vi "FGV Post Processing.vi"(4 "reprocessing index for filname":i32, 5 "LIN/EPA Refs Array":refnum<vi>[](array[refnum]), 6 "Aktion":T7, 7 "Refs Cluster":T3, 8 "error in (no error)":errorcluster caption="Fehler (Eingang, kein Fehler)", 9 "active Index Cluster in":T1, 10 "filenemas Cluster":T6, 11 "SpanInletClusterArray in":T8[](array[typedef]) {"zusätzliche Zeitdauer Erster Punkt" min=30 step=1 format="%#_5g"; "Zeitdauer Stufen" format="%#_5g"; "Max Fehler" format="%#_5g"; "Anzahl Stufen" format="%#_5g"; "Komponenten"."Komponente 5"."Komponente:" items=["NO (350,3000) LP 191C", "NO2 (150) LP 191C (1of2)", "NO2 (2000) LP 191C (2of2)", "N2O (300) LP 191C (1of2)", "NH3 (300) LP 191C (1of2)", "NH3 (900,3000) LP 191C (2of2)", "HNCO (400) 191C", "H2O% (30) LP 191C", "Formaldehyde (70,500) LP 191C", "CO2 low% (4) LP 191C (2of2)", "CO2% (20) LP 191C (1of2)", "CO (700) LP 191C (1of3)", "CO% (1) LP 191C (2of3)", "Propylene (1000) LP 191C", "Aromatic HC C7 (500) LP 191C", "Ethylene (1000) LP 191C", "CH4 (250) LP 191C (1of2)", "CH4 (5000) LP 191C (2of2)", "Ethane (1000) LP 191C", "Acetylene (1000) LP 191C", "HNO2 (20) 191C", "MeOH (1000) 191C", "CO% (10) LP 191C (3of3)", "Formic Acid (100) 191C", "SO2 (500) LP 191C", "Acetaldehyde (1000) LP 191C", "COS (100) LP 191C", "1,3 butadiene (100) LP 191C", "Oil as Octane (200) LP 191C", "N2O (1000) LP 191C (2of2)", "Propane (200) LP 191C", "NO2 autorange (2000)", "CO autorange (100000)", "CH4 autorange (5000)", "NH3 autorange (3000)", "Temp. Gascell", "Pressure Gascell", "sBeam@2500"]; "Komponenten"."Komponente 5"."Konzentration IST" format="%#.4f"; "Komponenten"."Komponente 5"."Genauigkeit" format="%#.1f"; "Komponenten"."Komponente 4"."Komponente:" items=["NO (350,3000) LP 191C", "NO2 (150) LP 191C (1of2)", "NO2 (2000) LP 191C (2of2)", "N2O (300) LP 191C (1of2)", "NH3 (300) LP 191C (1of2)", "NH3 (900,3000) LP 191C (2of2)", "HNCO (400) 191C", "H2O% (30) LP 191C", "Formaldehyde (70,500) LP 191C", "CO2 low% (4) LP 191C (2of2)", "CO2% (20) LP 191C (1of2)", "CO (700) LP 191C (1of3)", "CO% (1) LP 191C (2of3)", "Propylene (1000) LP 191C", "Aromatic HC C7 (500) LP 191C", "Ethylene (1000) LP 191C", "CH4 (250) LP 191C (1of2)", "CH4 (5000) LP 191C (2of2)", "Ethane (1000) LP 191C", "Acetylene (1000) LP 191C", "HNO2 (20) 191C", "MeOH (1000) 191C", "CO% (10) LP 191C (3of3)", "Formic Acid (100) 191C", "SO2 (500) LP 191C", "Acetaldehyde (1000) LP 191C", "COS (100) LP 191C", "1,3 butadiene (100) LP 191C", "Oil as Octane (200) LP 191C", "N2O (1000) LP 191C (2of2)", "Propane (200) LP 191C", "NO2 autorange (2000)", "CO autorange (100000)", "CH4 autorange (5000)", "NH3 autorange (3000)", "Temp. Gascell", "Pressure Gascell", "sBeam@2500"]; "Komponenten"."Komponente 4"."Konzentration IST" format="%#.4f"; "Komponenten"."Komponente 4"."Genauigkeit" format="%#.1f"; "Komponenten"."Komponente 3"."Komponente:" items=["NO (350,3000) LP 191C", "NO2 (150) LP 191C (1of2)", "NO2 (2000) LP 191C (2of2)", "N2O (300) LP 191C (1of2)", "NH3 (300) LP 191C (1of2)", "NH3 (900,3000) LP 191C (2of2)", "HNCO (400) 191C", "H2O% (30) LP 191C", "Formaldehyde (70,500) LP 191C", "CO2 low% (4) LP 191C (2of2)", "CO2% (20) LP 191C (1of2)", "CO (700) LP 191C (1of3)", "CO% (1) LP 191C (2of3)", "Propylene (1000) LP 191C", "Aromatic HC C7 (500) LP 191C", "Ethylene (1000) LP 191C", "CH4 (250) LP 191C (1of2)", "CH4 (5000) LP 191C (2of2)", "Ethane (1000) LP 191C", "Acetylene (1000) LP 191C", "HNO2 (20) 191C", "MeOH (1000) 191C", "CO% (10) LP 191C (3of3)", "Formic Acid (100) 191C", "SO2 (500) LP 191C", "Acetaldehyde (1000) LP 191C", "COS (100) LP 191C", "1,3 butadiene (100) LP 191C", "Oil as Octane (200) LP 191C", "N2O (1000) LP 191C (2of2)", "Propane (200) LP 191C", "NO2 autorange (2000)", "CO autorange (100000)", "CH4 autorange (5000)", "NH3 autorange (3000)", "Temp. Gascell", "Pressure Gascell", "sBeam@2500"]; "Komponenten"."Komponente 3"."Konzentration IST" format="%#.4f"; "Komponenten"."Komponente 3"."Genauigkeit" format="%#.1f"; "Komponenten"."Komponente 2"."Komponente:" items=["NO (350,3000) LP 191C", "NO2 (150) LP 191C (1of2)", "NO2 (2000) LP 191C (2of2)", "N2O (300) LP 191C (1of2)", "NH3 (300) LP 191C (1of2)", "NH3 (900,3000) LP 191C (2of2)", "HNCO (400) 191C", "H2O% (30) LP 191C", "Formaldehyde (70,500) LP 191C", "CO2 low% (4) LP 191C (2of2)", "CO2% (20) LP 191C (1of2)", "CO (700) LP 191C (1of3)", "CO% (1) LP 191C (2of3)", "Propylene (1000) LP 191C", "Aromatic HC C7 (500) LP 191C", "Ethylene (1000) LP 191C", "CH4 (250) LP 191C (1of2)", "CH4 (5000) LP 191C (2of2)", "Ethane (1000) LP 191C", "Acetylene (1000) LP 191C", "HNO2 (20) 191C", "MeOH (1000) 191C", "CO% (10) LP 191C (3of3)", "Formic Acid (100) 191C", "SO2 (500) LP 191C", "Acetaldehyde (1000) LP 191C", "COS (100) LP 191C", "1,3 butadiene (100) LP 191C", "Oil as Octane (200) LP 191C", "N2O (1000) LP 191C (2of2)", "Propane (200) LP 191C", "NO2 autorange (2000)", "CO autorange (100000)", "CH4 autorange (5000)", "NH3 autorange (3000)", "Temp. Gascell", "Pressure Gascell", "sBeam@2500"]; "Komponenten"."Komponente 2"."Konzentration IST" format="%#.4f"; "Komponenten"."Komponente 2"."Genauigkeit" format="%#.1f"; "Komponenten"."Komponente 1"."Komponente:" items=["NO (350,3000) LP 191C", "NO2 (150) LP 191C (1of2)", "NO2 (2000) LP 191C (2of2)", "N2O (300) LP 191C (1of2)", "NH3 (300) LP 191C (1of2)", "NH3 (900,3000) LP 191C (2of2)", "HNCO (400) 191C", "H2O% (30) LP 191C", "Formaldehyde (70,500) LP 191C", "CO2 low% (4) LP 191C (2of2)", "CO2% (20) LP 191C (1of2)", "CO (700) LP 191C (1of3)", "CO% (1) LP 191C (2of3)", "Propylene (1000) LP 191C", "Aromatic HC C7 (500) LP 191C", "Ethylene (1000) LP 191C", "CH4 (250) LP 191C (1of2)", "CH4 (5000) LP 191C (2of2)", "Ethane (1000) LP 191C", "Acetylene (1000) LP 191C", "HNO2 (20) 191C", "MeOH (1000) 191C", "CO% (10) LP 191C (3of3)", "Formic Acid (100) 191C", "SO2 (500) LP 191C", "Acetaldehyde (1000) LP 191C", "COS (100) LP 191C", "1,3 butadiene (100) LP 191C", "Oil as Octane (200) LP 191C", "N2O (1000) LP 191C (2of2)", "Propane (200) LP 191C", "NO2 autorange (2000)", "CO autorange (100000)", "CH4 autorange (5000)", "NH3 autorange (3000)", "Temp. Gascell", "Pressure Gascell", "sBeam@2500"]; "Komponenten"."Komponente 1"."Konzentration IST" format="%#.4f"; "Komponenten"."Komponente 1"."Genauigkeit" format="%#.1f"; "Ablaufdatum" format="%<%d.%m.%Y>T"; "Gasflasche" items=["----"=10000, "IAG NH3 3000"=0, "IAG NH3 200"=1, "IAG NH3 2000"=2, "IAG MG"=3, "IAG O2"=4]}) -> (0 "error out":errorcluster caption="Fehler (Ausgang)", 1 "active Index Cluster out":T2, 2 "filenemas Cluster Array":T5(array[cluster]), 3 "Index active SPANs":i32[](array[numeric]))   [LabVIEW 2020, in "Linearisierung v2.lvlib" / "SpanEinstellungen.lvlib"]
uses:
  SpanEinstellungen.lvlib
  SpanInletCluster.ctl
  Seiten/System Einstellungen V2/Konfig Gasflasche.ctl
  Seiten/System Einstellungen V2/Analysatoren.ctl
  Seiten/System Einstellungen V2/Gasflasche Auswahl.ctl
  Komponentencluster mit Formel.ctl
  Komponentenauswahl mit Formel.ctl
  Visualisierungs Elemente/String - Eingabefeld.ctl
  Einheit.ctl
  Seiten/System Einstellungen V2/Traegergas.ctl
  Aktion FGV Post Processing.ctl
  Visualisierungs Elemente/Pfad-Eingabefeld.ctl
  Postprocessing_Running_Indices.ctl
  Aktion FGV Spans abarbeiten.ctl
  <vilib>/Utility/miscctls.llb/LVStringsAndValuesArrayTypeDef_U16.ctl
  Aktion FGV SPAN Verriegelung.ctl
  Aktion FGV SpanEinstellungen.ctl
  Seiten/System Einstellungen V2/System Einstellungen V2.lvlib
panel:
  # "sec"
  # "%"
  # "sec"
  # "Komponente"
  # "Formel"
  # "Konzentration"
  # "Einheit"
  # "Genauigkeit [%]"
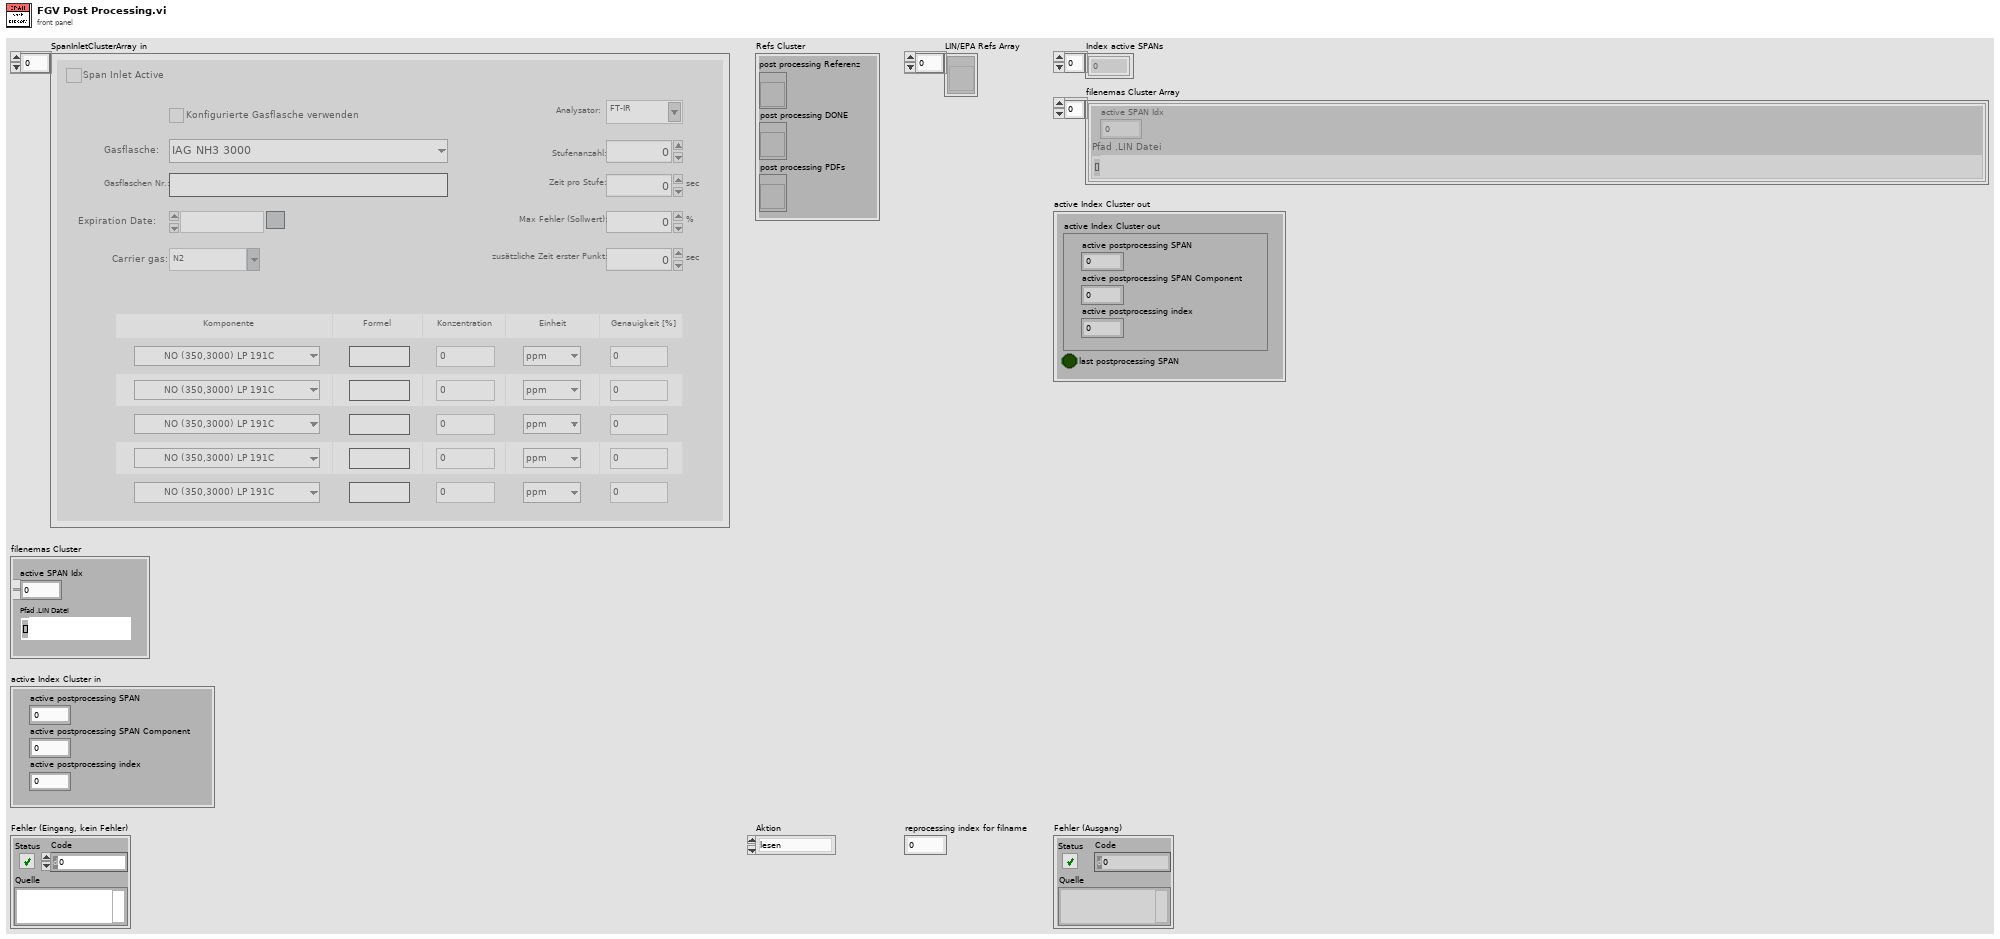
[diagram p1: front panel]
types:
  T1 = typedef "Linearisierung v2.lvlib/SpanEinstellungen.lvlib/Postprocessing_Running_Indices.ctl" = cluster{"active postprocessing SPAN":i32, "active postprocessing SPAN Component":i32, "active postprocessing index":i32}
  T2 = cluster{"active Index Cluster out":T1, "last postprocessing SPAN ":bool}
  T3 = cluster{"post processing Referenz":refnum<vi>, "post processing DONE":refnum<vi>, "post processing PDFs":refnum<vi>}
  T4 = typedef "Pfad-Eingabefeld.ctl" = path
  T5 = cluster{"active SPAN Idx":i32, "Pfad .LIN Datei":T4}[]
  T6 = cluster{"active SPAN Idx":i32, "Pfad .LIN Datei":T4}
  T7 = typedef "Linearisierung v2.lvlib/SpanEinstellungen.lvlib/Aktion FGV Post Processing.ctl" = enum16{"lesen", "set ref", "init", "reset", "enable", "disable", "filenames", "active", "comp", "filename index", "next", "first", "abort", "show", "same"}
  T8 = typedef "Linearisierung v2.lvlib/SpanEinstellungen.lvlib/SpanInletCluster.ctl" = cluster{"Span Inlet Active":T9, "Analysator":T10, "Konfig Gasflasche":T9, "Gasflasche":T11, "Gasflaschen Nr.:":string, "Ablaufdatum":timestamp, "Komponenten":T12, "Zeitdauer Stufen":sgl, "Max Fehler":sgl, "Anzahl Stufen":sgl, "Trägergas":T16, "zusätzliche Zeitdauer Erster Punkt":sgl}
  T9 = typedef "System Einstellungen V2.lvlib/Konfig Gasflasche.ctl" = bool
  T10 = typedef "System Einstellungen V2.lvlib/Analysatoren.ctl" = string
  T11 = typedef "System Einstellungen V2.lvlib/Gasflasche Auswahl.ctl" = u16
  T12 = typedef "Linearisierung v2.lvlib/SpanEinstellungen.lvlib/Komponentencluster mit Formel.ctl" = cluster{"Komponente 1":T13, "Komponente 2":T13, "Komponente 3":T13, "Komponente 4":T13, "Komponente 5":T13}
  T13 = typedef "Linearisierung v2.lvlib/SpanEinstellungen.lvlib/Komponentenauswahl mit Formel.ctl" = cluster{"Komponente:":u16, "Summenformel":T14, "Konzentration IST":dbl, "Einheit":T15, "Genauigkeit":dbl}
  T14 = typedef "String - Eingabefeld.ctl" = string
  T15 = typedef "Linearisierung v2.lvlib/SpanEinstellungen.lvlib/Einheit.ctl" = enum16{"ppm", "%"}
  T16 = typedef "System Einstellungen V2.lvlib/Traegergas.ctl" = string
  T17 = typedef "Linearisierung v2.lvlib/SpanEinstellungen.lvlib/Aktion FGV Spans abarbeiten.ctl" = enum16{"lesen", "idle", "start", "next", "comp", "init", "running", "abort"}
  T18 = typedef "LVStringsAndValuesArrayTypeDef_U16.ctl" = cluster{"String":string, "Value":u16}[]
  T19 = typedef "Linearisierung v2.lvlib/SpanEinstellungen.lvlib/Aktion FGV SPAN Verriegelung.ctl" = enum16{"lesen", "setrefs", "setcomp", "lock", "unlock", "Set Save EPA redirect", "Reset Save EPA redirect", "Set Postprocessing PDF", "Reset Postprocessing PDF", "Set Start Postprocessing PDF", "Reset Start Postprocessing PDF"}
  T20 = typedef "Linearisierung v2.lvlib/SpanEinstellungen.lvlib/Aktion FGV SpanEinstellungen.ctl" = enum16{"lesen", "schreiben", "laden", "speichern", "RegisterRef", "automatisch", "init", "PDF Params", "Punkte umkehren"}
  T21 = enum8{"Enabled", "Disabled", "Disabled and Grayed Out"}
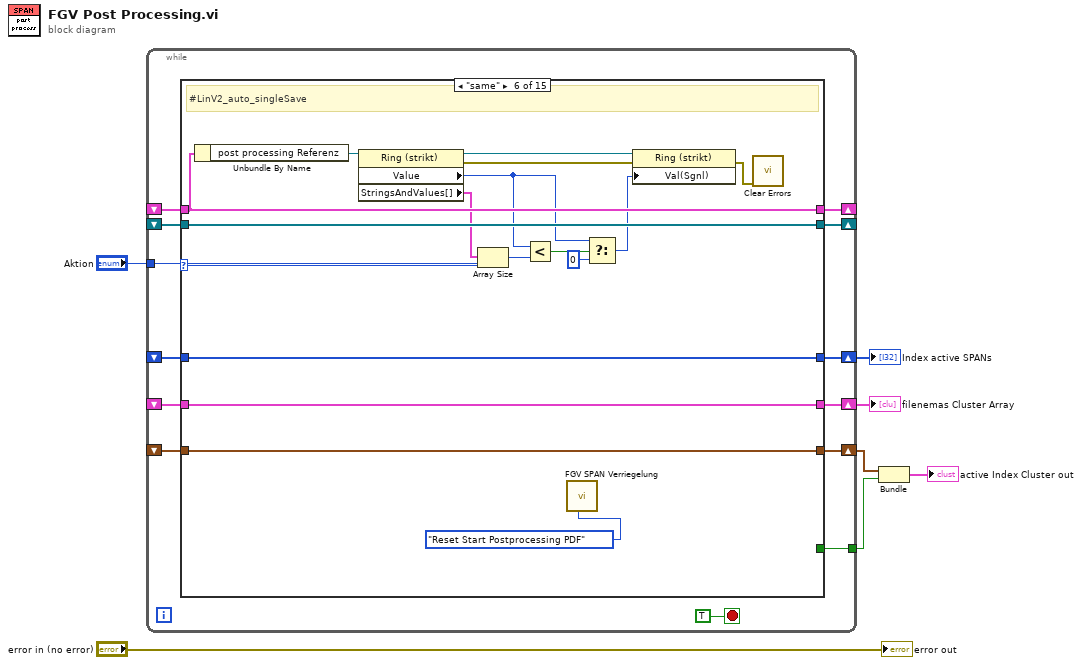
[diagram p0: block diagram]
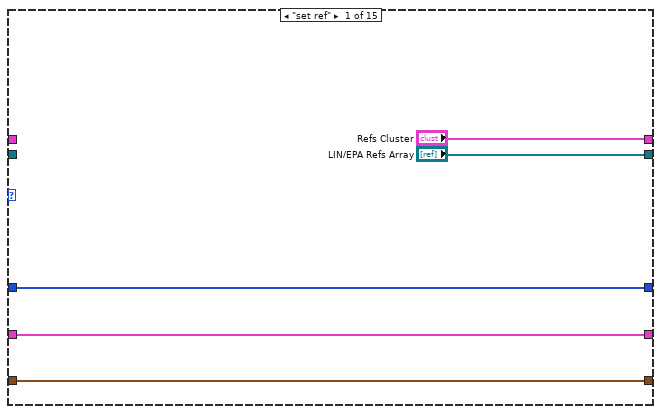
[diagram p2: hidden frame]
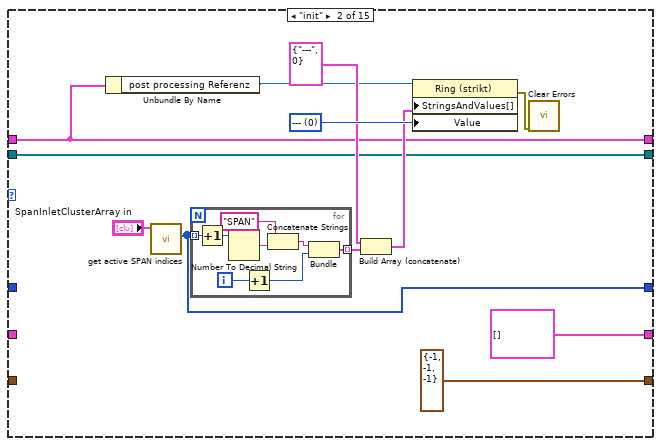
[diagram p3: hidden frame]
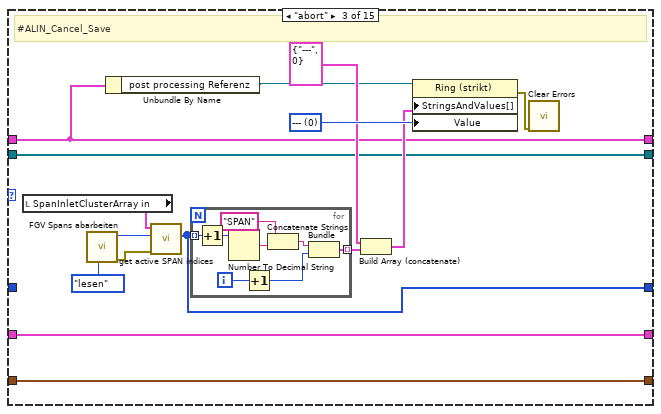
[diagram p4: hidden frame]
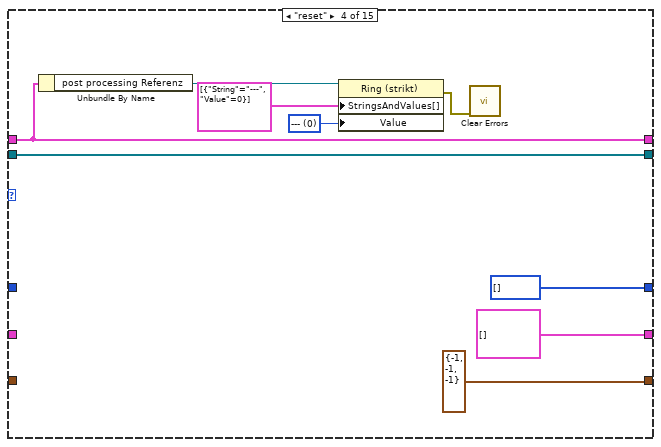
[diagram p5: hidden frame]
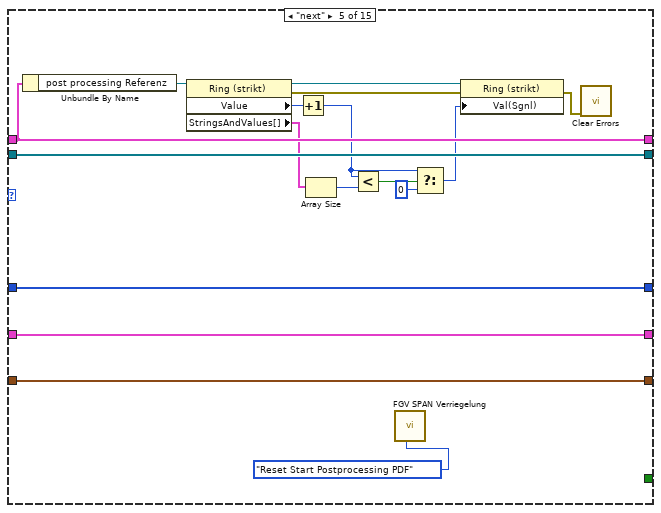
[diagram p6: hidden frame]
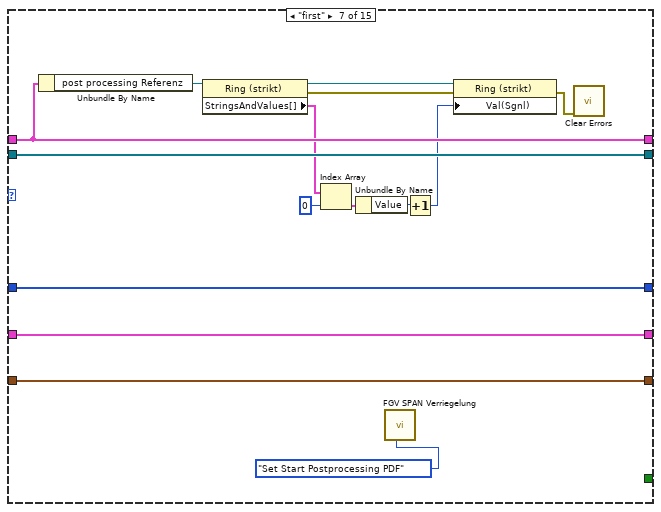
[diagram p7: hidden frame]
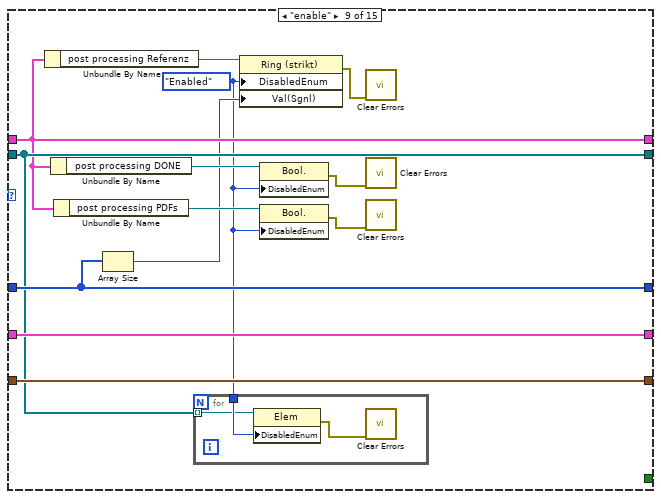
[diagram p9: hidden frame]
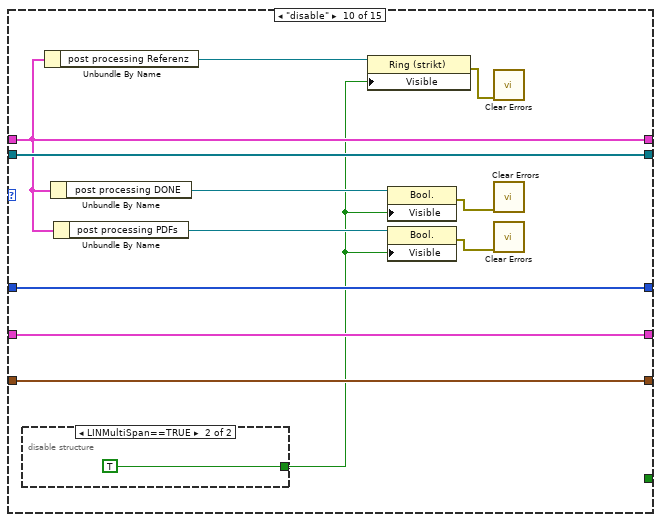
[diagram p10: hidden frame]
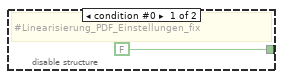
[diagram p11: hidden frame]
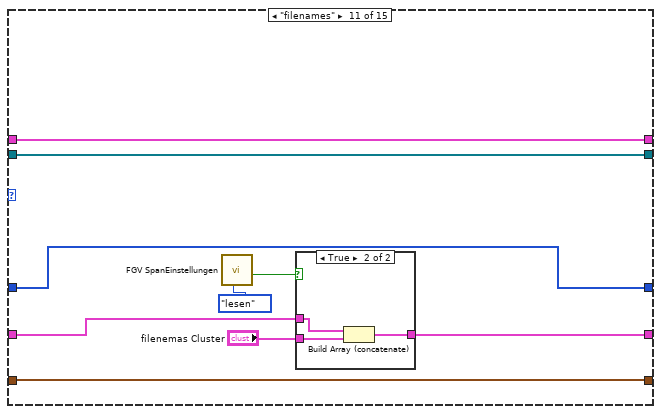
[diagram p12: hidden frame]
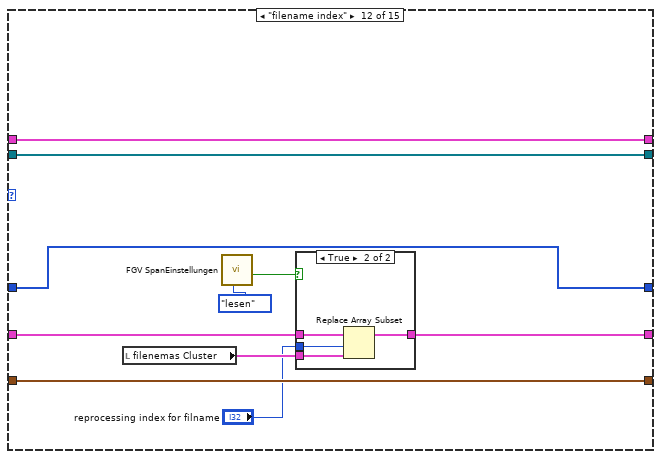
[diagram p14: hidden frame]
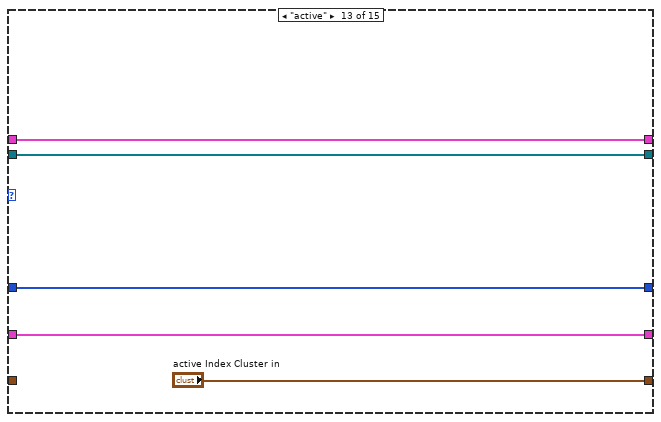
[diagram p16: hidden frame]
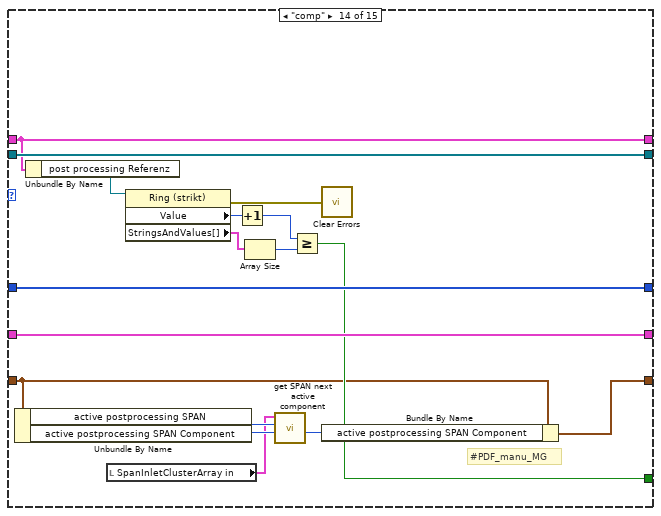
[diagram p17: hidden frame]
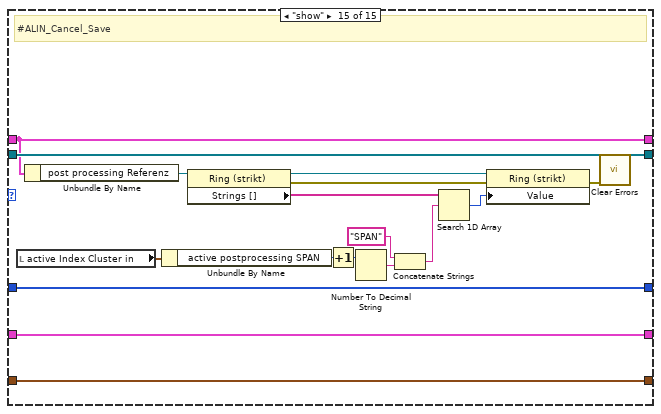
[diagram p18: hidden frame]
diagram:
  n1 = while {
    tunnel: "Aktion" -> [w20]
    shift-right: [w18] -> _
    shift-left: _ -> [w17]
    shift-right: [w16] -> w5
    shift-left: _ -> [w15]
    shift-right: [w14] -> w4
    shift-left: _ -> [w13]
    shift-right: [w8] -> w1
    shift-left: _ -> [w12]
    shift-right: [w11] -> _
    shift-left: _ -> [w10]
    tunnel: [w9] -> w3
    stop <- TRUE stop-if-true
    n2 = case shown="\"same\"" w20 {
      tunnel: ["Refs Cluster" w27 w53 w70 w93 w109 w124 w130 w133 w148 w169 w183 w193 w198 w223] -> w18
      tunnel: w17 -> [_ w27 w53 w70 w93 w109 w124 w130 w133 w148 w169 w183 w193 w198 w223]
      tunnel: [w25 T5 [] w50 T5 [] w86 w102 w118 w129 w142 w157 w165 w180 w192 w210 w227] -> w16
      tunnel: w15 -> [w25 _ w50 _ w86 w102 w118 w129 w142 w157 w164 w179 w192 w210 w227]
      tunnel: [w24 w32 w57 i32[] [] ("Index active SPAN") w87 w103 w119 w128 w137 w152 w163 w178 w191 w209 w226] -> w14
      tunnel: w13 -> [w24 _ _ _ w87 w103 w119 w128 w137 w152 w163 w178 w191 w209 w226]
      tunnel: [w23 T1 {"active postprocessing SPAN"=-1, "active postprocessing SPAN Component"=-1, "active postprocessing index"=-1} ("active Index Cluster in") w51 T1 {"active postprocessing SPAN"=-1, "active postprocessing SPAN Component"=-1, "active postprocessing index"=-1} ("active Index Cluster in") w85 w101 w117 w127 w141 w156 w162 w177 "active Index Cluster in" w196 w225] -> w8
      tunnel: w12 -> [w23 _ w51 _ w85 w101 w117 w127 w141 w156 w162 w177 _ w195 w225]
      tunnel: ["LIN/EPA Refs Array" w26 w52 w69 w92 w108 w123 w126 w136 w151 w161 w176 w189 w204 w224] -> w11
      tunnel: w10 -> [_ w26 w52 w69 w92 w108 w123 w126 w136 w151 w161 w176 w189 w204 w224]
      tunnel: [_ _ _ _ _ _ _ _ _ _ _ _ _ w197 _] -> w9
      frame "set ref" {
      }
      frame "init" {
        w34 = u16 0 items=["---", "NO (350,3000) LP 191C", "NO2 (150) LP 191C (1of2)", "NO2 (2000) LP 191C (2of2)", "N2O (300) LP 191C (1of2)", "NH3 (300) LP 191C (1of2)", "NH3 (900,3000) LP 191C (2of2)", "HNCO (400) 191C", "H2O% (30) LP 191C", "Formaldehyde (70,500) LP 191C", "CO2 low% (4) LP 191C (2of2)", "CO2% (20) LP 191C (1of2)", "CO (700) LP 191C (1of3)", "CO% (1) LP 191C (2of3)", "Propylene (1000) LP 191C", "Aromatic HC C7 (500) LP 191C", "Ethylene (1000) LP 191C", "CH4 (250) LP 191C (1of2)", "CH4 (5000) LP 191C (2of2)", "Ethane (1000) LP 191C", "Acetylene (1000) LP 191C", "HNO2 (20) 191C", "MeOH (1000) 191C", "CO% (10) LP 191C (3of3)", "Formic Acid (100) 191C", "SO2 (500) LP 191C", "Acetaldehyde (1000) LP 191C", "COS (100) LP 191C", "1,3 butadiene (100) LP 191C", "Oil as Octane (200) LP 191C", "N2O (1000) LP 191C (2of2)", "Propane (200) LP 191C", "NO2 autorange (2000)", "CO autorange (100000)", "CH4 autorange (5000)", "NH3 autorange (3000)", "NOx autorange (3000)", "HCD (10000)", "NMHCD (10000)", "CO2% autorange (20)", "H2Oppm (300000)", "N2O autorange (1000)", "NMNEHCD (3000)", "Temp. Gascell", "Pressure Gascell", "sBeam@2500", "Temp. HL zu FT-IR", "Temp. HL Extern SP1", "Austrittstemp. FT-IR", "Temp. Schaltschrank", "Konstant 0", "Konstant 50", "Konstant 100", "AK DUMMY"] ("post processing")
        n3 = Unbundle By Name(w27) -> ("post processing Referenz"=w28:refnum<vi>)
        n4 = call "get active SPAN indices.vi"("SpanInletClusterArray in"="SpanInletClusterArray in") -> ("Index active SPAN"=w32:i32[])  [unwired: 8 in, 2 out]
        n5 = for {
          tunnel: w32 -> [w44] mode=indexing
          tunnel: [w43] -> w35 mode=indexing
          i -> [w40]
          n6 = Increment(x=w44) -> (x+1=w38:i32)
          n7 = Number To Decimal String(number=w38) -> (decimal integer string=w45:string)  [unwired: 1 in]
          n8 = Increment(x=w40) -> (x+1=w39:i32)
          n9 = Concatenate Strings("SPAN" ("String"), w45) -> (w42:string)
          n10 = Bundle(w42, w39) -> (w43:cluster{string, i32})  [unwired: 1 in]
        }
        n11 = Build Array (concatenate)(cluster{"String":string, "Value":u16} {"String"="---", "Value"=0} ("Strings und Werte []"), w35) -> (w31:cluster{"String":string, "Value":i32}[])
        n12 = property class="Ring (strikt)"(reference=w28, "StringsAndValues[]"=w31, "Value"=w34) -> (error out=w36:errorcluster)  [unwired: 1 in, 1 out]
        n13 = call <vilib>:"Clear Errors.vi"("error in (no error)"=w36) -> ()  [unwired: 5 in, 2 out]
      }
      frame "abort" {
        w58 = u16 0 items=["---", "NO (350,3000) LP 191C", "NO2 (150) LP 191C (1of2)", "NO2 (2000) LP 191C (2of2)", "N2O (300) LP 191C (1of2)", "NH3 (300) LP 191C (1of2)", "NH3 (900,3000) LP 191C (2of2)", "HNCO (400) 191C", "H2O% (30) LP 191C", "Formaldehyde (70,500) LP 191C", "CO2 low% (4) LP 191C (2of2)", "CO2% (20) LP 191C (1of2)", "CO (700) LP 191C (1of3)", "CO% (1) LP 191C (2of3)", "Propylene (1000) LP 191C", "Aromatic HC C7 (500) LP 191C", "Ethylene (1000) LP 191C", "CH4 (250) LP 191C (1of2)", "CH4 (5000) LP 191C (2of2)", "Ethane (1000) LP 191C", "Acetylene (1000) LP 191C", "HNO2 (20) 191C", "MeOH (1000) 191C", "CO% (10) LP 191C (3of3)", "Formic Acid (100) 191C", "SO2 (500) LP 191C", "Acetaldehyde (1000) LP 191C", "COS (100) LP 191C", "1,3 butadiene (100) LP 191C", "Oil as Octane (200) LP 191C", "N2O (1000) LP 191C (2of2)", "Propane (200) LP 191C", "NO2 autorange (2000)", "CO autorange (100000)", "CH4 autorange (5000)", "NH3 autorange (3000)", "NOx autorange (3000)", "HCD (10000)", "NMHCD (10000)", "CO2% autorange (20)", "H2Oppm (300000)", "N2O autorange (1000)", "NMNEHCD (3000)", "Temp. Gascell", "Pressure Gascell", "sBeam@2500", "Temp. HL zu FT-IR", "Temp. HL Extern SP1", "Austrittstemp. FT-IR", "Temp. Schaltschrank", "Konstant 0", "Konstant 50", "Konstant 100", "AK DUMMY"] ("post processing")
        # "#ALIN_Cancel_Save"
        n14 = local read "SpanInletClusterArray in"() -> (w49:T8[])
        n15 = call "FGV Spans abarbeiten.vi"("Aktion"=Aktion_FGV_Spans_abarbeiten."lesen") -> ("error out"=w46:errorcluster, "active SPAN Idx out"=w47:i32)  [unwired: 5 in, 4 out]
        n16 = Unbundle By Name(w53) -> ("post processing Referenz"=w54:refnum<vi>)
        n17 = call "get active SPAN indices.vi"("error in (no error)"=w46, "max active SPAN Idx in"=w47, "SpanInletClusterArray in"=w49) -> ("Index active SPAN"=w57:i32[])  [unwired: 6 in, 2 out]
        n18 = for {
          tunnel: w57 -> [w67] mode=indexing
          tunnel: [w66] -> w59 mode=indexing
          i -> [w63]
          n19 = Increment(x=w67) -> (x+1=w61:i32)
          n20 = Number To Decimal String(number=w61) -> (decimal integer string=w68:string)  [unwired: 1 in]
          n21 = Increment(x=w63) -> (x+1=w62:i32)
          n22 = Concatenate Strings("SPAN" ("String"), w68) -> (w65:string)
          n23 = Bundle(w65, w62) -> (w66:cluster{string, i32})  [unwired: 1 in]
        }
        n24 = Build Array (concatenate)(cluster{"String":string, "Value":u16} {"String"="---", "Value"=0} ("Strings und Werte []"), w59) -> (w56:cluster{"String":string, "Value":i32}[])
        n25 = property class="Ring (strikt)"(reference=w54, "StringsAndValues[]"=w56, "Value"=w58) -> (error out=w60:errorcluster)  [unwired: 1 in, 1 out]
        n26 = call <vilib>:"Clear Errors.vi"("error in (no error)"=w60) -> ()  [unwired: 5 in, 2 out]
      }
      frame "reset" {
        w76 = u16 0 items=["---", "NO (350,3000) LP 191C", "NO2 (150) LP 191C (1of2)", "NO2 (2000) LP 191C (2of2)", "N2O (300) LP 191C (1of2)", "NH3 (300) LP 191C (1of2)", "NH3 (900,3000) LP 191C (2of2)", "HNCO (400) 191C", "H2O% (30) LP 191C", "Formaldehyde (70,500) LP 191C", "CO2 low% (4) LP 191C (2of2)", "CO2% (20) LP 191C (1of2)", "CO (700) LP 191C (1of3)", "CO% (1) LP 191C (2of3)", "Propylene (1000) LP 191C", "Aromatic HC C7 (500) LP 191C", "Ethylene (1000) LP 191C", "CH4 (250) LP 191C (1of2)", "CH4 (5000) LP 191C (2of2)", "Ethane (1000) LP 191C", "Acetylene (1000) LP 191C", "HNO2 (20) 191C", "MeOH (1000) 191C", "CO% (10) LP 191C (3of3)", "Formic Acid (100) 191C", "SO2 (500) LP 191C", "Acetaldehyde (1000) LP 191C", "COS (100) LP 191C", "1,3 butadiene (100) LP 191C", "Oil as Octane (200) LP 191C", "N2O (1000) LP 191C (2of2)", "Propane (200) LP 191C", "NO2 autorange (2000)", "CO autorange (100000)", "CH4 autorange (5000)", "NH3 autorange (3000)", "NOx autorange (3000)", "HCD (10000)", "NMHCD (10000)", "CO2% autorange (20)", "H2Oppm (300000)", "N2O autorange (1000)", "NMNEHCD (3000)", "Temp. Gascell", "Pressure Gascell", "sBeam@2500", "Temp. HL zu FT-IR", "Temp. HL Extern SP1", "Austrittstemp. FT-IR", "Temp. Schaltschrank", "Konstant 0", "Konstant 50", "Konstant 100", "AK DUMMY"] ("post processing")
        n27 = Unbundle By Name(w70) -> ("post processing Referenz"=w71:refnum<vi>)
        n28 = property class="Ring (strikt)"(reference=w71, "StringsAndValues[]"=T18 [{"String"="---", "Value"=0}] ("Strings und Werte []"), "Value"=w76) -> (error out=w75:errorcluster)  [unwired: 1 in, 1 out]
        n29 = call <vilib>:"Clear Errors.vi"("error in (no error)"=w75) -> ()  [unwired: 5 in, 2 out]
      }
      frame "next" {
        n30 = Unbundle By Name(w93) -> ("post processing Referenz"=w94:refnum<vi>)
        n31 = property class="Ring (strikt)"(reference=w94) -> (reference out=w90:refnum<vi>, error out=w91:errorcluster, "Value"=w88:u16, "StringsAndValues[]"=w84:T18)  [unwired: 1 in]
        n32 = Increment(x=w88) -> (x+1=w80:u16)
        n33 = Array Size(array=w84) -> (size(s)=w83:i32)
        n34 = Less?(x=w80, y=w83) -> (x < y?=w82:bool)
        n35 = call "FGV SPAN Verriegelung.vi"("aktion"=Aktion_FGV_SPAN_Verriegelung."Reset Start Postprocessing PDF") -> ()  [unwired: 8 in, 3 out]
        n36 = Select(t=w80, s=w82, f=u16 0 ("t")) -> (s? t:f=w81:u16)
        n37 = property class="Ring (strikt)"(reference=w90, error in=w91, "Val(Sgnl)"=w81) -> (error out=w89:errorcluster)  [unwired: 1 out]
        n38 = call <vilib>:"Clear Errors.vi"("error in (no error)"=w89) -> ()  [unwired: 5 in, 2 out]
      }
      frame "same" {
        # "#LinV2_auto_singleSave"
        n39 = Unbundle By Name(w109) -> ("post processing Referenz"=w110:refnum<vi>)
        n40 = property class="Ring (strikt)"(reference=w110) -> (reference out=w106:refnum<vi>, error out=w107:errorcluster, "Value"=w104:u16, "StringsAndValues[]"=w100:T18)  [unwired: 1 in]
        n41 = Array Size(array=w100) -> (size(s)=w99:i32)
        n42 = Less?(x=w104, y=w99) -> (x < y?=w98:bool)
        n43 = call "FGV SPAN Verriegelung.vi"("aktion"=Aktion_FGV_SPAN_Verriegelung."Reset Start Postprocessing PDF") -> ()  [unwired: 8 in, 3 out]
        n44 = Select(t=w104, s=w98, f=u16 0 ("t")) -> (s? t:f=w97:u16)
        n45 = property class="Ring (strikt)"(reference=w106, error in=w107, "Val(Sgnl)"=w97) -> (error out=w105:errorcluster)  [unwired: 1 out]
        n46 = call <vilib>:"Clear Errors.vi"("error in (no error)"=w105) -> ()  [unwired: 5 in, 2 out]
      }
      frame "first" {
        n47 = Unbundle By Name(w124) -> ("post processing Referenz"=w125:refnum<vi>)
        n48 = property class="Ring (strikt)"(reference=w125) -> (reference out=w121:refnum<vi>, error out=w122:errorcluster, "StringsAndValues[]"=w116:T18)  [unwired: 1 in]
        n49 = Index Array(array=w116, index=0 ("Index")) -> (element=w114:cluster{"String":string, "Value":u16})
        n50 = Unbundle By Name(w114) -> ("Value"=w113:u16)
        n51 = call "FGV SPAN Verriegelung.vi"("aktion"=Aktion_FGV_SPAN_Verriegelung."Set Start Postprocessing PDF") -> ()  [unwired: 8 in, 3 out]
        n52 = Increment(x=w113) -> (x+1=w112:u16)
        n53 = property class="Ring (strikt)"(reference=w121, error in=w122, "Val(Sgnl)"=w112) -> (error out=w120:errorcluster)  [unwired: 1 out]
        n54 = call <vilib>:"Clear Errors.vi"("error in (no error)"=w120) -> ()  [unwired: 5 in, 2 out]
      }
      frame "lesen", Default {
      }
      frame "enable" {
        w131 = T21."Enabled" ("Deaktiviert")
        n55 = Unbundle By Name(w133) -> ("post processing Referenz"=w140:refnum<vi>)
        n56 = Unbundle By Name(w133) -> ("post processing DONE"=w139:refnum<vi>)
        n57 = Unbundle By Name(w133) -> ("post processing PDFs"=w134:refnum<vi>)
        n58 = Array Size(array=w137) -> (size(s)=w132:i32)
        n59 = for {
          tunnel: w131 -> [w146]
          tunnel: w136 -> [w144] mode=indexing
          n60 = property class="Elem"(reference=w144, "DisabledEnum"=w146) -> (error out=w145:errorcluster)  [unwired: 1 in, 1 out]
          n61 = call <vilib>:"Clear Errors.vi"("error in (no error)"=w145) -> ()  [unwired: 5 in, 2 out]
        }
        n62 = property class="Ring (strikt)"(reference=w140, "DisabledEnum"=w131, "Val(Sgnl)"=w132) -> (error out=w143:errorcluster)  [unwired: 1 in, 1 out]
        n63 = property class="Bool."(reference=w139, "DisabledEnum"=w131) -> (error out=w138:errorcluster)  [unwired: 1 in, 1 out]
        n64 = property class="Bool."(reference=w134, "DisabledEnum"=w131) -> (error out=w135:errorcluster)  [unwired: 1 in, 1 out]
        n65 = call <vilib>:"Clear Errors.vi"("error in (no error)"=w143) -> ()  [unwired: 5 in, 2 out]
        n66 = call <vilib>:"Clear Errors.vi"("error in (no error)"=w138) -> ()  [unwired: 5 in, 2 out]
        n67 = call <vilib>:"Clear Errors.vi"("error in (no error)"=w135) -> ()  [unwired: 5 in, 2 out]
      }
      frame "disable" {
        n68 = disable-structure shown="LINMultiSpan==TRUE" {
          disable-tunnel: [FALSE TRUE] -> w147
          frame condition #0 {
            # "#Linearisierung_PDF_Einstellungen_fix"
          }
          frame condition #1 (active) {
          }
        }
        n69 = Unbundle By Name(w148) -> ("post processing Referenz"=w155:refnum<vi>)
        n70 = Unbundle By Name(w148) -> ("post processing DONE"=w154:refnum<vi>)
        n71 = Unbundle By Name(w148) -> ("post processing PDFs"=w149:refnum<vi>)
        n72 = property class="Ring (strikt)"(reference=w155, "Visible"=w147) -> (error out=w158:errorcluster)  [unwired: 1 in, 1 out]
        n73 = property class="Bool."(reference=w154, "Visible"=w147) -> (error out=w153:errorcluster)  [unwired: 1 in, 1 out]
        n74 = property class="Bool."(reference=w149, "Visible"=w147) -> (error out=w150:errorcluster)  [unwired: 1 in, 1 out]
        n75 = call <vilib>:"Clear Errors.vi"("error in (no error)"=w158) -> ()  [unwired: 5 in, 2 out]
        n76 = call <vilib>:"Clear Errors.vi"("error in (no error)"=w153) -> ()  [unwired: 5 in, 2 out]
        n77 = call <vilib>:"Clear Errors.vi"("error in (no error)"=w150) -> ()  [unwired: 5 in, 2 out]
      }
      frame "filenames" {
        n78 = call "FGV SpanEinstellungen.vi"("Aktion"=Aktion_FGV_SpanEinstellungen."lesen") -> ("automatisch out"=w167:T9)  [unwired: 6 in, 4 out]
        n79 = case shown="True" w167 {
          tunnel: "filenemas Cluster" -> [_ w173]
          tunnel: [w170 w172] -> w165
          tunnel: w164 -> [w170 w171]
          frame False {
          }
          frame True {
            n80 = Build Array (concatenate)(w171, w173) -> (w172:T5)
          }
        }
      }
      frame "filename index" {
        n81 = local read "filenemas Cluster"() -> (w175:T6)
        n82 = call "FGV SpanEinstellungen.vi"("Aktion"=Aktion_FGV_SpanEinstellungen."lesen") -> ("automatisch out"=w181:T9)  [unwired: 6 in, 4 out]
        n83 = case shown="True" w181 {
          tunnel: w175 -> [_ w186]
          tunnel: [w184 w188] -> w180
          tunnel: w179 -> [w184 w187]
          tunnel: "reprocessing index for filname" -> [_ w185]
          frame False {
          }
          frame True {
            n84 = Replace Array Subset(array=w187, new element=w186, index=w185) -> (w188:T5)
          }
        }
      }
      frame "active" {
      }
      frame "comp" {
        # "#PDF_manu_MG"
        n85 = Unbundle By Name(w195) -> ("active postprocessing SPAN"=w208:i32, "active postprocessing SPAN Component"=w207:i32)
        n86 = Unbundle By Name(w198) -> ("post processing Referenz"=w203:refnum<vi>)
        n87 = local read "SpanInletClusterArray in"() -> (w205:T8[])
        n88 = property class="Ring (strikt)"(reference=w203) -> (error out=w194:errorcluster, "Value"=w202:u16, "StringsAndValues[]"=w201:T18)  [unwired: 1 in, 1 out]
        n89 = Increment(x=w202) -> (x+1=w199:u16)
        n90 = Array Size(array=w201) -> (size(s)=w200:i32)
        n91 = call "get SPAN next active component.vi"("Komponente Idx"=w207, "SPAN Idx"=w208, "SpanInletClusterArray in"=w205) -> ("next aktive Komponente"=w206:i32)  [unwired: 6 in, 2 out]
        n92 = Greater Or Equal?(x=w199, y=w200) -> (x >= y?=w197:bool)
        n93 = call <vilib>:"Clear Errors.vi"("error in (no error)"=w194) -> ()  [unwired: 5 in, 2 out]
        n94 = Bundle By Name(cluster=w195, "active postprocessing SPAN Component"=w206) -> (w196:T1)
      }
      frame "show" {
        # "#ALIN_Cancel_Save"
        n95 = local read "active Index Cluster in"() -> (w221:T1)
        n96 = Unbundle By Name(w223) -> ("post processing Referenz"=w220:refnum<vi>)
        n97 = Unbundle By Name(w221) -> ("active postprocessing SPAN"=w215:i32)
        n98 = property class="Ring (strikt)"(reference=w220) -> (reference out=w219:refnum<vi>, error out=w218:errorcluster, "Strings []"=w214:string[])  [unwired: 1 in]
        n99 = Increment(x=w215) -> (x+1=w211:i32)
        n100 = Number To Decimal String(number=w211) -> (decimal integer string=w217:string)  [unwired: 1 in]
        n101 = Concatenate Strings("SPAN" ("String"), w217) -> (w213:string)
        n102 = Search 1D Array(1D array=w214, element=w213) -> (index of element=w212:i32)  [unwired: 1 in]
        n103 = property class="Ring (strikt)"(reference=w219, error in=w218, "Value"=w212) -> (error out=w222:errorcluster)  [unwired: 1 out]
        n104 = call <vilib>:"Clear Errors.vi"("error in (no error)"=w222) -> ()  [unwired: 5 in, 2 out]
      }
    }
  }
  "filenemas Cluster Array" <- w5
  "Index active SPANs" <- w4
  n105 = Bundle("active Index Cluster in"=w1, w3) -> (→"active Index Cluster out":cluster{"active Index Cluster in":T1, bool})  [unwired: 1 in]
  "error out" <- "error in (no error)"
